vi "RasterScan.vi"() -> ()   [LabVIEW 2009]
panel:
  out "Ring Text.Text":string
  out "Final Y":dbl
  out "Final X":dbl
  out "Start Y":dbl=53210.0
  out "Start X":dbl=24018.0
  out "Raster Scan":dbl[][](graph)
  in  "Step":dbl=10.0
  in  "Size":i32=5
  in  "Actuator":enum16{"AERO-ME"}(ring)
  in  "Sensor":enum16{"NICMOS"}(ring)
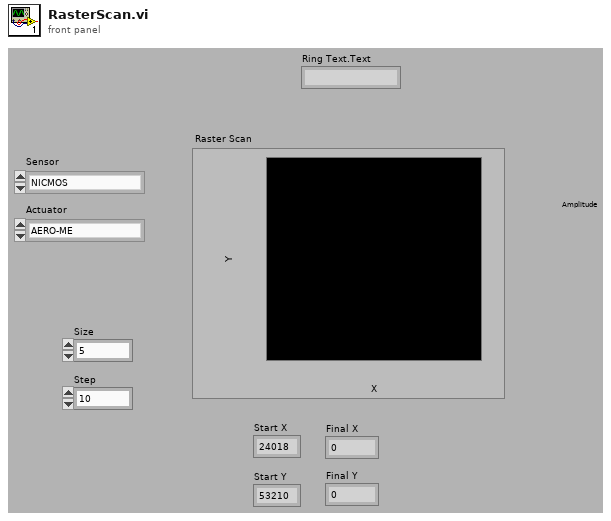
[diagram p1: front panel]
types:
  T1 = enum16{"Acquire", "GetAbsolutePosition", "AbsoluteMove", "Release"}
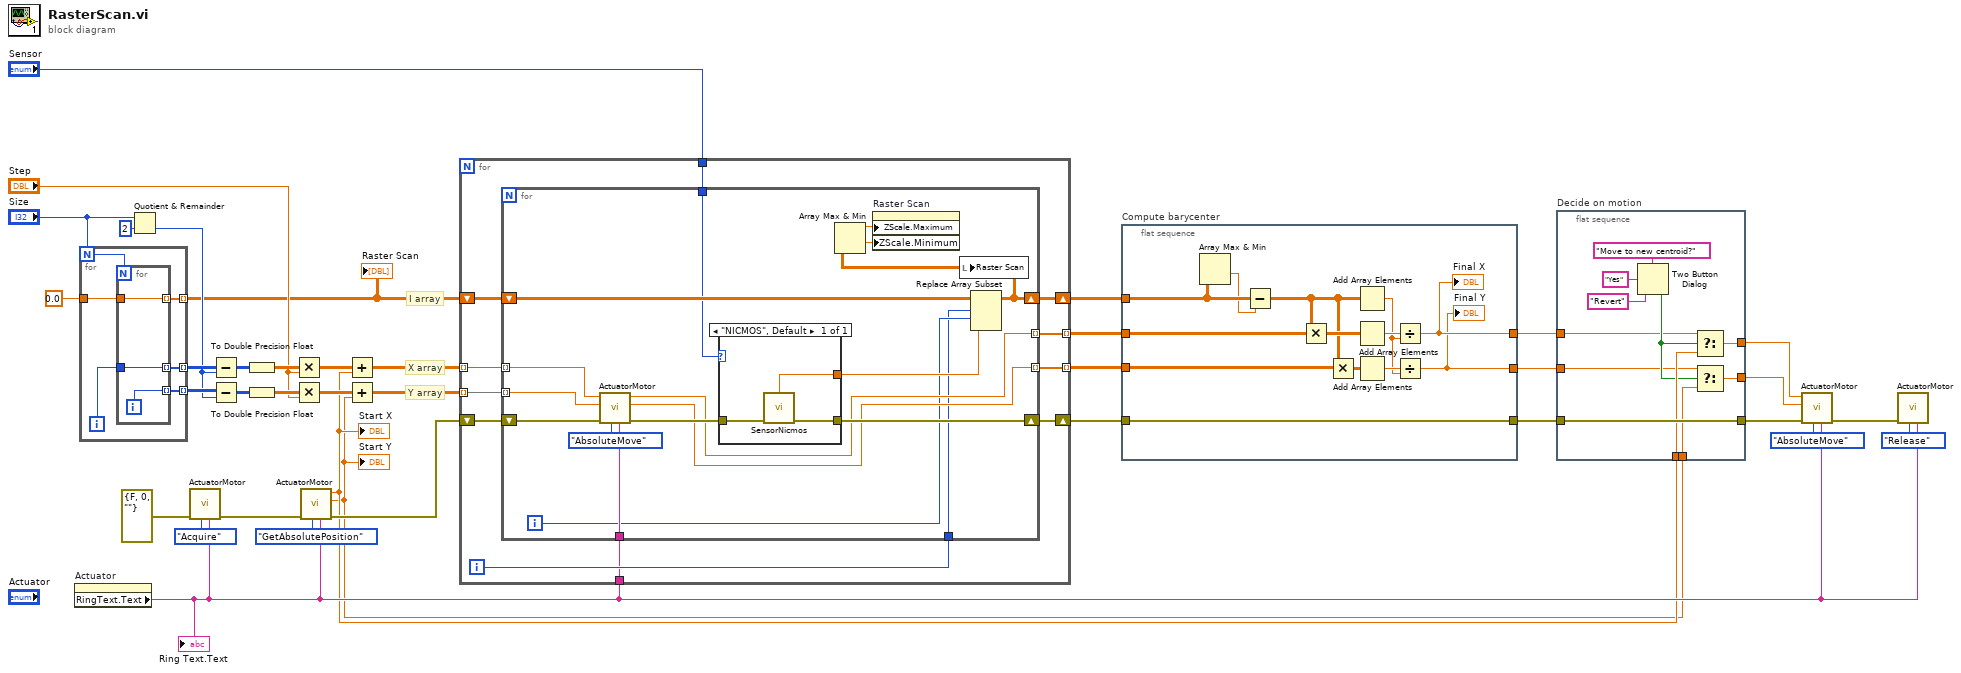
[diagram p0: block diagram]
diagram:
  # "I array"
  # "Y array"
  # "X array"
  n1 = property on="Actuator" class="Enum (strict)"() -> ("RingText.Text"=w11:string)  [unwired: 2 in, 2 out]
  "Ring Text.Text" <- w11
  n2 = for {
    N: "Size" -> [w41]
    tunnel: [w44] -> w38 mode=indexing
    tunnel: [w42] -> w37 mode=indexing
    tunnel: 0.0 ("element") -> [w40]
    tunnel: [w39] -> w4 mode=indexing
    i -> [w43]
    n3 = for {
      N: w41 -> [_]
      tunnel: [w47] -> w44 mode=indexing
      tunnel: w43 -> [w47]
      tunnel: [w46] -> w42 mode=indexing
      tunnel: w40 -> [w45]
      tunnel: [w45] -> w39 mode=indexing
      i -> [w46]
    }
  }
  "Raster Scan" <- w4
  n4 = Quotient & Remainder(x="Size", y=2) -> (floor(x/y)=w34:i32)  [unwired: 1 out]
  n5 = call "ActuatorMotor.vi"("Actuator Name"=w11, "Command"=T1."Acquire", "error in (no error)"=errorcluster {"status"=FALSE, "code"=0, "source"=""}) -> ("error out"=w20:errorcluster)  [unwired: 4 in, 2 out]
  n6 = Subtract(x=w38, y=w34) -> (x-y=w32:i32[][])
  n7 = Subtract(x=w37, y=w34) -> (x-y=w29:i32[][])
  n8 = To Double Precision Float(number=w32) -> (double precision float=w31:dbl[][])
  n9 = To Double Precision Float(number=w29) -> (double precision float=w30:dbl[][])
  n10 = Multiply(x=w31, y="Step") -> (x*y=w18:dbl[][])
  n11 = Multiply(x=w30, y="Step") -> (x*y=w16:dbl[][])
  n12 = call "ActuatorMotor.vi"("Actuator Name"=w11, "Command"=T1."GetAbsolutePosition", "error in (no error)"=w20) -> ("error out"=w24:errorcluster, "Y out"=w7:dbl, "X out"=w8:dbl)  [unwired: 4 in]
  "Start X" <- w8
  "Start Y" <- w7
  n13 = Add(x=w18, y=w8) -> (x+y=w17:dbl[][])
  n14 = Add(x=w16, y=w7) -> (x+y=w15:dbl[][])
  n15 = for {
    tunnel: w17 -> [w58] mode=indexing
    tunnel: w15 -> [w57] mode=indexing
    shift-right: [w48] -> w3
    shift-left: w4 -> [w56]
    tunnel: "Sensor" -> [w53]
    shift-right: [w52] -> w26
    shift-left: w24 -> [w54]
    tunnel: [w51] -> w23 mode=indexing
    tunnel: [w50] -> w22 mode=indexing
    tunnel: w11 -> [w49]
    i -> [w55]
    n16 = for {
      tunnel: w58 -> [w68] mode=indexing
      tunnel: w57 -> [w67] mode=indexing
      shift-right: [w63] -> w48
      shift-left: w56 -> [w75]
      tunnel: w55 -> [w59]
      tunnel: w53 -> [w73]
      shift-right: [w70] -> w52
      shift-left: w54 -> [w72]
      tunnel: [w66] -> w51 mode=indexing
      tunnel: [w65] -> w50 mode=indexing
      tunnel: w49 -> [w64]
      i -> [w60]
      n17 = call "ActuatorMotor.vi"("Actuator Name"=w64, "Command"=T1."AbsoluteMove", "error in (no error)"=w72, "Y"=w67, "X"=w68) -> ("error out"=w71:errorcluster, "Y out"=w65:dbl, "X out"=w66:dbl)  [unwired: 2 in]
      n18 = case shown="\"NICMOS\", Default" w73 {
        tunnel: [w78] -> w74
        tunnel: w71 -> [w77]
        tunnel: [w76] -> w70
        frame "NICMOS", Default {
          n19 = call "SensorNicmos.vi"("error in (no error)"=w77) -> ("error out"=w76:errorcluster, "Intensity"=w78:dbl)  [unwired: 3 in]
        }
      }
      n20 = Replace Array Subset(array=w75, new element=w74, index (row)=w59, index (col)=w60) -> (w63:dbl[][])
      n21 = Array Max & Min(array=w63) -> (max value=w62:dbl, min value=w61:dbl)  [unwired: 2 out]
      n22 = property on="Raster Scan" class="IntGraph (strict)"("ZScale.Maximum"=w62, "ZScale.Minimum"=w61) -> ()  [unwired: 2 in, 2 out]
      n23 = local write "Raster Scan"(w63) -> ()
    }
  }
  n24 = flat-sequence "Compute barycenter" {
    tunnel: w26 -> [w91]
    tunnel: [w91] -> w10
    tunnel: w23 -> [w90]
    tunnel: w22 -> [w89]
    tunnel: w3 -> [w83]
    tunnel: [w80] -> w2
    tunnel: [w79] -> w1
    frame #0 {
      n25 = Array Max & Min(array=w83) -> (min value=w81:dbl)  [unwired: 3 out]
      n26 = Subtract(x=w83, y=w81) -> (x-y=w82:dbl[][])
      n27 = Multiply(x=w82, y=w90) -> (x*y=w88:dbl[][])
      n28 = Multiply(x=w82, y=w89) -> (x*y=w87:dbl[][])
      n29 = Add Array Elements(numeric array=w82) -> (sum=w84:dbl)
      n30 = Add Array Elements(numeric array=w88) -> (sum=w86:dbl)
      n31 = Add Array Elements(numeric array=w87) -> (sum=w85:dbl)
      n32 = Divide(x=w86, y=w84) -> (x/y=w80:dbl)
      "Final X" <- w80
      n33 = Divide(x=w85, y=w84) -> (x/y=w79:dbl)
      "Final Y" <- w79
    }
  }
  n34 = flat-sequence "Decide on motion" {
    tunnel: w10 -> [w99]
    tunnel: [w99] -> w9
    tunnel: w8 -> [w95]
    tunnel: w7 -> [w96]
    tunnel: [w98] -> w6
    tunnel: [w97] -> w5
    tunnel: w2 -> [w93]
    tunnel: w1 -> [w92]
    frame #0 {
      n35 = Two Button Dialog(message="Move to new centroid?", 1:"Revert" ("F button name (\"Cancel\")"), 2:"Yes" ("T button name (\"OK\")")) -> (T button?=w94:bool)
      n36 = Select(t=w93, s=w94, f=w95) -> (s? t:f=w98:dbl)
      n37 = Select(t=w92, s=w94, f=w96) -> (s? t:f=w97:dbl)
    }
  }
  n38 = call "ActuatorMotor.vi"("Actuator Name"=w11, "Command"=T1."AbsoluteMove", "error in (no error)"=w9, "Y"=w5, "X"=w6) -> ("error out"=w12:errorcluster)  [unwired: 2 in, 2 out]
  n39 = call "ActuatorMotor.vi"("Actuator Name"=w11, "Command"=T1."Release", "error in (no error)"=w12) -> ()  [unwired: 4 in, 3 out]
